vi "editscenario Load Scenario.vi"(6 "User Information":T1, 7 "command (\"edit\")":string="edit", 8 "error in (no error)":errorcluster, 9 "CONTENT (\"\")":string, 10 "sxScenarioId (\"\")":string, 11 "Connection Refnum":T3) -> (0 "error out":errorcluster, 1 "Template Keys":T2, 2 "sxScenarioId":string, 3 "Connection Refnum":T3, 5 "PREVSCENARIOS array":string)   [LabVIEW 2011]
uses:
  Summitek EXT/ODBC/SQL Controls/Connection Refnum.ctl
  ITK EXT/utils/keyedarr.llb/Keyed Array.ctl
  server/database/Users/User Record.ctl
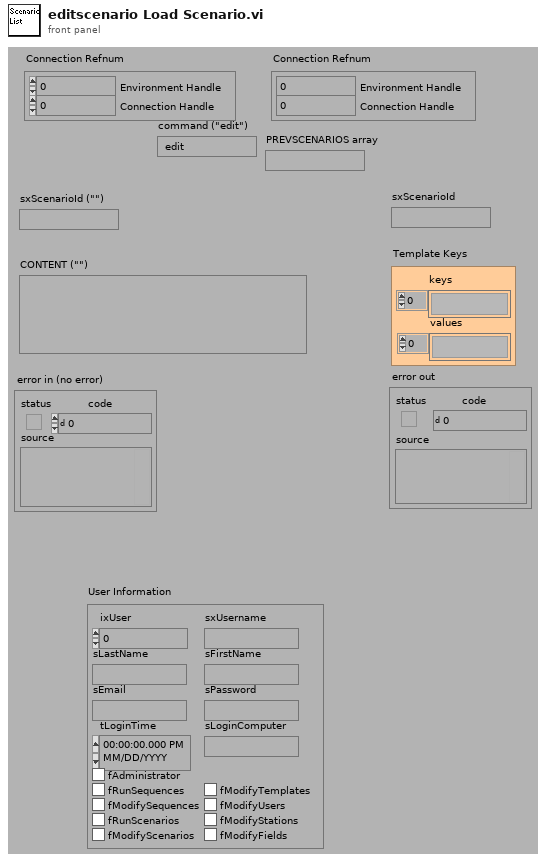
[diagram p1: front panel]
types:
  T1 = typedef "User Record.ctl" = cluster{"ixUser":i32, "sxUsername":string, "sLastName":string, "sFirstName":string, "sEmail":string, "sPassword":string, "tLoginTime":timestamp, "sLoginComputer":string, "fAdministrator":bool, "fRunSequences":bool, "fModifySequences":bool, "fRunScenarios":bool, "fModifyScenarios":bool, "fModifyTemplates":bool, "fModifyUsers":bool, "fModifyStations":bool, "fModifyFields":bool}
  T2 = typedef "Keyed Array.ctl" = cluster{"keys":string[], "values":string[]}
  T3 = typedef "Connection Refnum.ctl" = cluster{"Environment Handle":i32, "Connection Handle":i32}
  T4 = typedef "Scenario Record.ctl" = cluster{"ixScenario":i32, "tCreated":timestamp, "tModified":timestamp, "sxUsername":string, "sModifiedBy":string, "sxScenarioId":string, "sDescription":string, "sLogic":string, "sResultFieldsCSV":string, "sTemplatesCSV":string, "fAutoRunReports":bool, "fSortByTemplates":bool, "fCombinePDF":bool, "Conditions":T5[]}
  T5 = typedef "Condition Record.ctl" = cluster{"iConditionIndex":i32, "sxFieldId":string, "nOperator":T6, "sMatchValue":string}
  T6 = typedef "Condition Operators.ctl" = enum16{"equal (=)", "not equal (\\u2260)", "less than (<)", "less than or equal (\\u2264)", "greater than (>)", "greater than or equal (\\u2265)", "contains", "does not contain"}
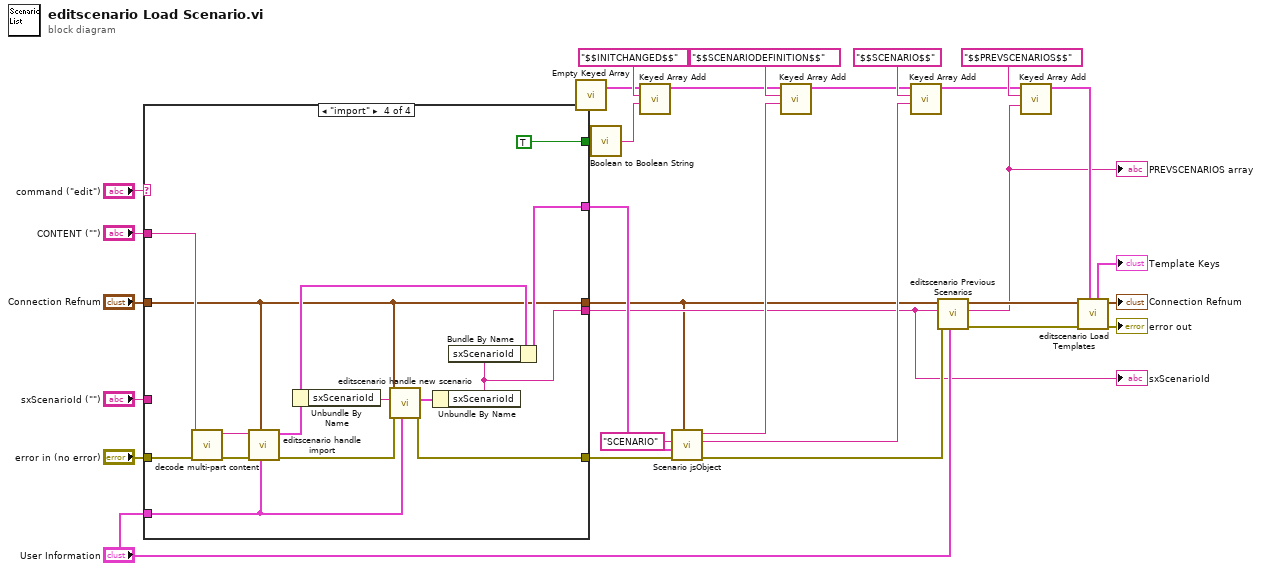
[diagram p0: block diagram]
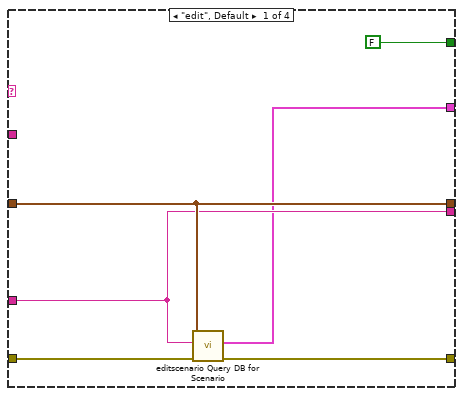
[diagram p2: hidden frame]
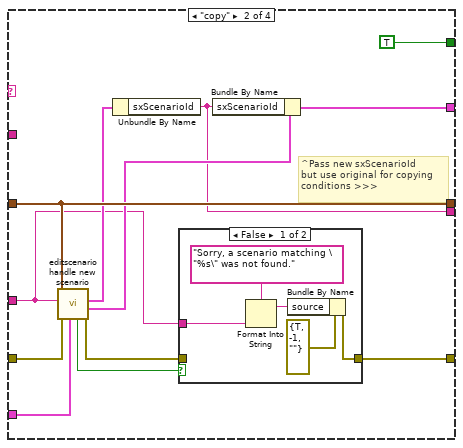
[diagram p3: hidden frame]
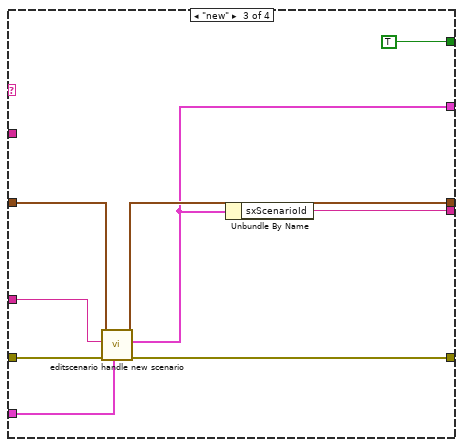
[diagram p5: hidden frame]
diagram:
  n1 = case shown="\"import\"" "command (\"edit\")" {
    tunnel: [w35 w49 w59 w74] -> w12
    tunnel: "sxScenarioId (\"\")" -> [w33 w39 w56 _]
    tunnel: "error in (no error)" -> [w36 w47 w63 w70]
    tunnel: "Connection Refnum" -> [w34 w44 w61 w65]
    tunnel: [w34 w44 w60 w65] -> w1
    tunnel: "User Information" -> [_ w42 w62 w76]
    tunnel: [FALSE TRUE TRUE TRUE] -> w24
    tunnel: [w32 w40 w58 w71] -> w16
    tunnel: [w33 w38 w57 w72] -> w4
    tunnel: "CONTENT (\"\")" -> [_ _ _ w68]
    frame "edit", Default {
      n2 = call "editscenario Query DB for Scenario.vi"("error in (no error)"=w36, "sxScenarioId (\"\")"=w33, "Connection Refnum"=w34) -> ("error out"=w35:errorcluster, "Scenario Record"=w32:T4)  [unwired: 7 out]
    }
    frame "copy" {
      # "^Pass new sxScenarioId\nbut use original for copying\nconditions >>>"
      n3 = call "editscenario handle new scenario.vi"("User Information"=w42, "error in (no error)"=w47, "New Name Suggestion\n(empty - \"Username Sequence N\")"=w39, "Connection Refnum"=w44) -> ("error out"=w45:errorcluster, "First Matching Scenario Record"=w43:T4, "New Scenario Record"=w41:T4, "Existed?"=w46:bool)  [unwired: 4 out]
      n4 = Unbundle By Name(w41) -> ("sxScenarioId"=w38:string)
      n5 = case shown="False" w46 {
        tunnel: w45 -> [_ w55]
        tunnel: [w51 w55] -> w49
        tunnel: w39 -> [w50 _]
        frame False {
          n6 = Format Into String(format string="Sorry, a scenario matching \"%s\" was not found.", w50) -> (resulting string=w53:string)  [unwired: 2 in, 1 out]
          n7 = Bundle By Name(cluster=errorcluster {"status"=TRUE, "code"=-1, "source"=""} ("error out"), "source"=w53) -> (w51:errorcluster)
        }
        frame True {
        }
      }
      n8 = Bundle By Name(cluster=w43, "sxScenarioId"=w38) -> (w40:T4)
    }
    frame "new" {
      n9 = call "editscenario handle new scenario.vi"("User Information"=w62, "error in (no error)"=w63, "New Name Suggestion\n(empty - \"Username Sequence N\")"=w56, "Connection Refnum"=w61) -> ("error out"=w59:errorcluster, "New Scenario Record"=w58:T4, "Connection Refnum"=w60:T3)  [unwired: 5 out]
      n10 = Unbundle By Name(w58) -> ("sxScenarioId"=w57:string)
    }
    frame "import" {
      n11 = call "decode multi-part content.vi"("error in (no error)"=w70, "Multi-Part Content (\"\")"=w68) -> ("error out"=w69:errorcluster, "Content"=w67:string)  [unwired: 1 in, 7 out]
      n12 = call "editscenario handle import.vi"("User Information"=w76, "Connection Refnum"=w65, "error in (no error)"=w69, "Scenario XML (\"\")"=w67) -> ("error out"=w77:errorcluster, "Scenario Record"=w66:T4)  [unwired: 1 in, 5 out]
      n13 = Unbundle By Name(w66) -> ("sxScenarioId"=w75:string)
      n14 = call "editscenario handle new scenario.vi"("User Information"=w76, "error in (no error)"=w77, "New Name Suggestion\n(empty - \"Username Sequence N\")"=w75, "Connection Refnum"=w65) -> ("error out"=w74:errorcluster, "New Scenario Record"=w73:T4)  [unwired: 6 out]
      n15 = Unbundle By Name(w73) -> ("sxScenarioId"=w72:string)
      n16 = Bundle By Name(cluster=w66, "sxScenarioId"=w72) -> (w71:T4)
    }
  }
  "sxScenarioId" <- w4
  n17 = call "Empty Keyed Array.vi"() -> ("empty keyed array"=w3:T2)  [unwired: 3 out]
  n18 = call "Boolean to Boolean String.vi"("Boolean"=w24) -> ("Boolean string"=w25:string)  [unwired: 1 in]
  n19 = call "Keyed Array Add.vi"("value"=w25, "key"="$$INITCHANGED$$", "array in"=w3) -> ("array out"=w18:T2)  [unwired: 1 in, 3 out]
  n20 = call "Scenario jsObject.vi"("Connection Refnum"=w1, "error in (no error)"=w12, "Scenario Record (empty)"=w16, "Scenario jsObject Name (\"\")"="SCENARIO" ("Scenario jsObject Name (\"\")")) -> ("error out"=w7:errorcluster, "Scenario jsObject"=w14:string, "SCENARIO jsObject Definition"=w15:string)  [unwired: 2 in, 3 out]
  n21 = call "Keyed Array Add.vi"("value"=w15, "key"="$$SCENARIODEFINITION$$", "array in"=w18) -> ("array out"=w17:T2)  [unwired: 1 in, 3 out]
  n22 = call "Keyed Array Add.vi"("value"=w14, "key"="$$SCENARIO$$", "array in"=w17) -> ("array out"=w10:T2)  [unwired: 1 in, 3 out]
  n23 = call "editscenario Previous Scenarios.vi"("User Information"="User Information", "error in (no error)"=w7, "sxScenarioId (\"\")"=w4, "Connection Refnum"=w1) -> ("error out"=w8:errorcluster, "Previous SCENARIOS array"=w5:string, "Connection Refnum"=w6:T3)  [unwired: 1 in, 4 out]
  "PREVSCENARIOS array" <- w5
  n24 = call "Keyed Array Add.vi"("value"=w5, "key"="$$PREVSCENARIOS$$", "array in"=w10) -> ("array out"=w9:T2)  [unwired: 1 in, 3 out]
  n25 = call "editscenario Load Templates.vi"("Template Keys (empty)"=w9, "error in (no error)"=w8, "Connection Refnum"=w6) -> ("error out"=→"error out":errorcluster, "Connection Refnum"=→"Connection Refnum":T3, "Template Keys"=→"Template Keys":T2)  [unwired: 6 out]
